vi "SaveOffsets.vi"(2 "error in":errorcluster, 3 "CAN Talon SRX Ref":T1[](array[typedef]), 4 "configuration file path":path) -> (0 "error out":errorcluster)   [LabVIEW 2016, in "Team900SwerveDrive.lvlib"]
uses:
  Team900SwerveDrive.lvlib
  <vilib>/Rock Robotics/WPI/MotorControl/WPI_MotorControlDeviceRef.ctl
  <vilib>/Rock Robotics/WPI/MotorControl/WPI_MotorControlType.ctl
  <vilib>/Rock Robotics/SystemInterfaces/DIO/FPGA_DIOPWMChannel.ctl
  <vilib>/Rock Robotics/WPI/PWM/WPI_PWMDeadband.ctl
  <vilib>/Utility/config.llb/Write Key (Double).vi
  SwerveGlobalData.vi
  <vilib>/Utility/config.llb/NI_LVConfig.lvlib
panel:
  # "Assumes the wheels are all at their zero position\n(pointed directly to the right of the robot, such\nthat if the speed motors were run with positive\nthrottle the robot would move right), and uses\nthese sensor positions to save the offsets in a\nconfig file"
  # "Thought: since config files can be edited directly\nthrough the roboRIO webdash, this is largely\nunnecessary"
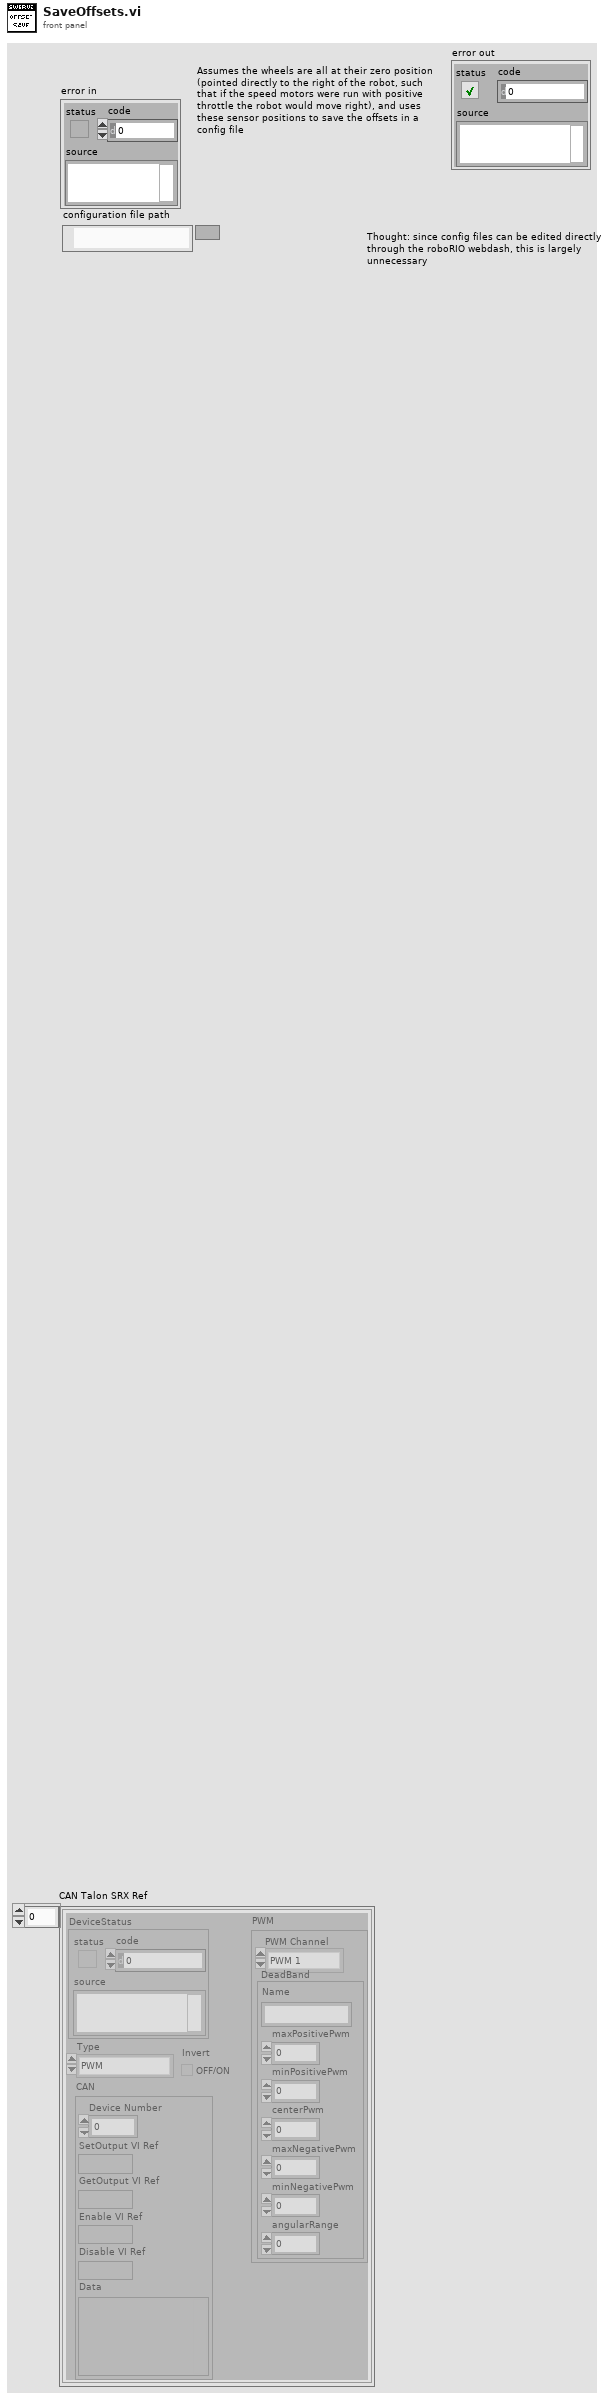
[diagram p1: front panel]
types:
  T1 = typedef "WPI_MotorControlDeviceRef.ctl" = cluster{"DeviceStatus":errorcluster, "Type":T2, "PWM":cluster{"PWM Channel":T3, "DeadBand":T4}, "CAN":cluster{"Device Number":u8, "SetOutput VI Ref":variant, "GetOutput VI Ref":variant, "Enable VI Ref":variant, "Disable VI Ref":variant, "Data":variant}, "Invert":bool}
  T2 = typedef "WPI_MotorControlType.ctl" = enum16{"PWM", "CAN"}
  T3 = typedef "FPGA_DIOPWMChannel.ctl" = enum8{"PWM 0", "PWM 1", "PWM 2", "PWM 3", "PWM 4", "PWM 5", "PWM 6", "PWM 7", "PWM 8", "PWM 9", "PWM MXP 0", "PWM MXP 1", "PWM MXP 2", "PWM MXP 3", "PWM MXP 4", "PWM MXP 5", "PWM MXP 6", "PWM MXP 7", "PWM MXP 8", "PWM MXP 9", "Invalid"}
  T4 = typedef "WPI_PWMDeadband.ctl" = cluster{"Name":string, "maxPositivePwm":i32, "minPositivePwm":i32, "centerPwm":i32, "maxNegativePwm":i32, "minNegativePwm":i32, "angularRange":u16}
  T5 = typedef "WPI_CANTalonSRX_GlobalStatus.ctl" = cluster{"Applied Throttle":dbl, "Module Enabled":bool, "CAN Error":errorcluster, "Closed Loop Error":dbl, "Forward Limit Switch Closed":bool, "Reverse Limit Switch Closed":bool, "Sensor Position":dbl, "Sensor Velocity":dbl, "Current":dbl, "Sticky Fault - Over Temp":bool, "Sticky Fault - Under Voltage":bool, "Sticky Fault - Forward Limit":bool, "Sticky Fault - Reverse Limit":bool, "Sticky Fault - Forward Soft Limit":bool, "Sticky Fault - Reverse Soft Limit":bool, "Brake is Enabled":bool, "Encoder Position":dbl, "Encoder Velocity":dbl, "Encoder Index Count":dbl, "Encoder A Pin State":bool, "Encoder B Pin State":bool, "Encoder Index Pin State":bool, "Analog In":dbl, "Analog In Velocity":dbl, "Temperature (C)":dbl, "Battery Voltage":dbl, "Control 5 Is Supported":bool, "Current Profile Slot Select":dbl, "Pos Div 8":bool, "Vel Div 4":bool, "Pulse Width Position":i32, "Pulse Width Velocity":i32, "Pulse Width Rise To Rise (us)":i32, "Pulse Width Rise To Fall (us)":i32, "Mot Prof Active Is Under Run":bool, "Mot Prof Active Has Under Run":bool, "Mot Prof Active Is Last":bool, "Mot Prof Active Velocity Only":bool, "Mot Prof Active Is Valid":bool, "Mot Prof Buffer Is Full":bool, "Mot Prof Active Profile Slot Select":i32, "Mot Prof NextID":i32, "Mot Prof Count":i32, "Mot Prof Active Velocity":dbl, "Mot Prof Active Position":dbl, "Mot Prof Output Enable":i32}
  T6 = typedef "NI_LVConfig.lvlib/Config Data RefNum.ctl" = refnum<k1>
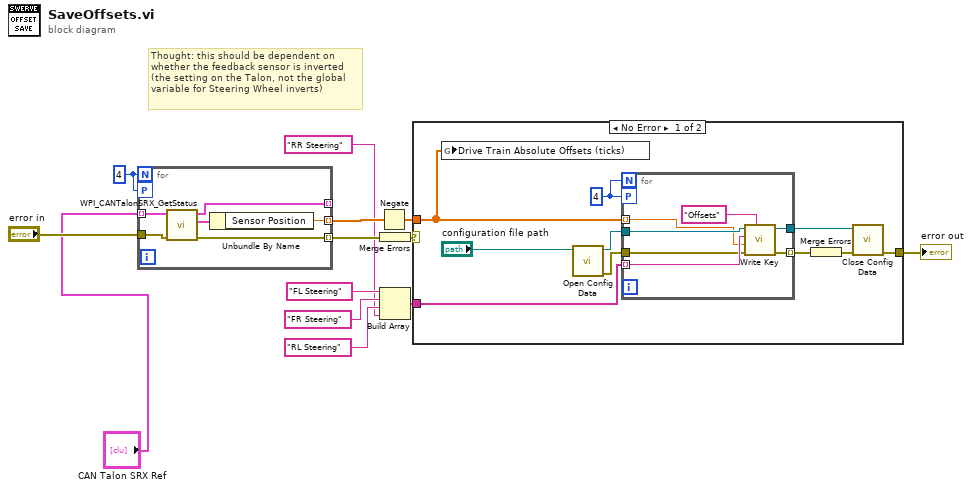
[diagram p0: block diagram]
diagram:
  w12 = 4
  # "Thought: this should be dependent on \nwhether the feedback sensor is inverted\n(the setting on the Talon, not the global\nvariable for Steering Wheel inverts)"
  n1 = for {
    N: w12 -> [_]
    tunnel: [w19] -> w10 mode=indexing
    tunnel: [w15] -> _ mode=indexing
    tunnel: "error in" -> [w17]
    tunnel: [w16] -> w11 mode=indexing
    workers-P: w12 -> [_]
    tunnel: "CAN Talon SRX Ref" -> [w14] mode=indexing
    n2 = call <vilib>:"WPI_CANTalonSRX_GetStatus.vi"("error in (no error)"=w17, "CAN Talon SRX Ref"=w14) -> ("error out"=w16:errorcluster, "Talon SRX Status"=w18:T5, "CAN Talon SRX Ref"=w15:T1)  [unwired: 7 in]
    n3 = Unbundle By Name(w18) -> ("Sensor Position"=w19:dbl)
  }
  n4 = Negate(x=w10) -> (-x=w9:dbl[])
  n5 = Merge Errors(w11) -> (w13:errorcluster)
  n6 = Build Array("FL Steering", "FR Steering" ("element"), "RL Steering" ("element"), "RR Steering" ("element")) -> (w4:string[])
  n7 = case shown="No Error" w13 {
    selector: w13 -> [_ w37]
    tunnel: w9 -> [w27 _]
    tunnel: w4 -> [w28 _]
    tunnel: [w20 w37] -> w3
    frame No Error {
      w29 = 4
      n8 = global write "SwerveGlobalData.vi" "Drive Train Absolute Offsets (ticks)"(w27) -> ()
      n9 = call <vilib>:"Open Config Data.vi"("configuration file path"="configuration file path") -> ("error out"=w23:errorcluster, "refnum"=w25:T6)  [unwired: 2 in, 7 out]
      n10 = for {
        N: w29 -> [_]
        tunnel: w25 -> [w36]
        workers-P: w29 -> [_]
        tunnel: w28 -> [w35] mode=indexing
        tunnel: w27 -> [w34] mode=indexing
        tunnel: [w33] -> w26 mode=indexing
        tunnel: w23 -> [w31]
        tunnel: [w30] -> w21
        n11 = call-poly <vilib>:"Write Key.vi"("section"="Offsets", "error in (no error)"=w31, "value"=w34, "key"=w35, "refnum"=w36) -> ("error out"=w33:errorcluster, "refnum out"=w30:T6)  [unwired: 3 in, 2 out]
      }
      n12 = Merge Errors(w26) -> (w22:errorcluster)
      n13 = call <vilib>:"Close Config Data.vi"("error in (no error)"=w22, "refnum"=w21) -> ("error out"=w20:errorcluster)  [unwired: 8 in, 1 out]
    }
    frame Error {
    }
  }
  "error out" <- w3
